vi "Launcher.vi"() -> ()   [LabVIEW 2023, in "Test Caller Actor.lvlib"]
uses:
  Test Caller Actor.lvlib
  Test Caller Actor/Test Caller Actor.lvclass
  Class Loader/Class Loader/Class Loader.lvclass
  Test Caller Actor/Test Caller Actor.lvclass/Test Caller Actor.ctl
  <vilib>/ActorFramework/Message Enqueuer/Message Enqueuer.lvclass/Message Enqueuer.ctl
  Test Caller Actor/Write Class Loader Enqueuer.vi
  <vilib>/ActorFramework/Message Enqueuer/Enqueue.vi
  <vilib>/ActorFramework/Stop Msg/Stop Msg.lvclass
  <vilib>/Utility/LVClass/Get LV Class Name.vi
  <resource>/AFDebug/Generate Trace for Message.vi
  <vilib>/ActorFramework/Message Priority Queue/Priority Enqueue.vi
  <vilib>/ActorFramework/Actor/Actor.lvclass
  C:/Program Files/National Instruments/LabVIEW 2023/vi.lib/LS Instruments AG/Async Methods Actor/Async Methods Actor/Async Methods Actor/Async Methods Actor.lvclass
  C:/Program Files/National Instruments/LabVIEW 2023/vi.lib/ActorFramework/Actor/Actor.lvclass
  C:/Projects/Shared Libraries/Class Loader/Class Loader/Class Loader/Class Loader.lvclass
  C:/Projects/Shared Libraries/Class Loader/Test Caller Actor/Test Caller Actor/Test Caller Actor.lvclass
  C:/Projects/Shared Libraries/Class Loader/Class Loader/Class Loader Interfaces/Class Loader Interfaces/Class Loader Interfaces.lvclass
panel:
  in  "Test Actor Number":i32=2
  in  "Stop Class Loader":bool
  out "error out":errorcluster
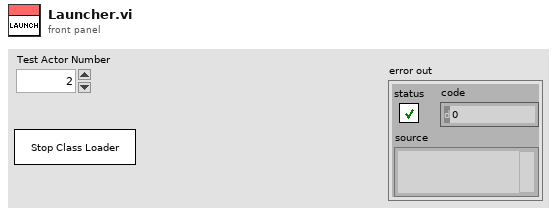
[diagram p1: front panel]
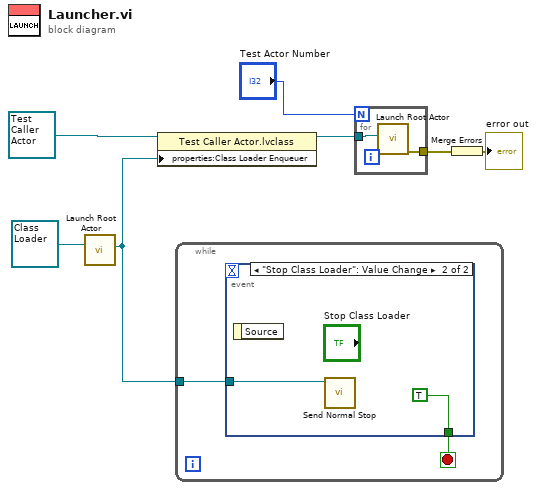
[diagram p0: block diagram]
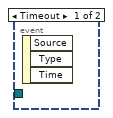
[diagram p2: hidden frame]
diagram:
  n1 = call <vilib>:"Launch Root Actor.vi"("Actor"=refnum<class "Class Loader.lvclass"> refnum ("Class Loader.lvlib:Class Loader.lvclass")) -> ("Actor's Enqueuer"=w2:refnum<class "Message Enqueuer.lvclass">)  [unwired: 9 in, 1 out]
  n2 = property class="Test Caller Actor.lvclass"(reference=refnum<class "Test Caller Actor.lvclass"> refnum ("Test Caller Actor.lvlib:Test Caller Actor.lvclass"), "properties:Class Loader Enqueuer"=w2) -> (reference out=w3:refnum<class "Test Caller Actor.lvclass">)  [unwired: 1 in, 1 out]
  n3 = while {
    tunnel: w2 -> [w9]
    stop <- w8 stop-if-true
    n4 = event shown="[1] \"Stop Class Loader\": Value Change" {
      selector: _ -> [_ _]
      dyn-events: _ -> [_ _]
      timeout: _ -> [_ _]
      tunnel: w9 -> [_ w11]
      tunnel: [_ TRUE] -> w8
      event Timeout {
        n5 = event-data() -> ()  [unwired: 1 in, 3 out]
      }
      event "Stop Class Loader": Value Change {
        n6 = event-data() -> ()  [unwired: 1 in, 1 out]
        n7 = call <vilib>:"Send Normal Stop.vi"("Message Enqueuer"=w11) -> ()  [unwired: 10 in, 1 out]
      }
    }
  }
  n8 = for {
    N: "Test Actor Number" -> [_]
    tunnel: [w13] -> w7
    tunnel: w3 -> [w12]
    n9 = call <vilib>:"Launch Root Actor.vi"("Actor"=w12) -> ("error out"=w13:errorcluster)  [unwired: 9 in, 1 out]
  }
  n10 = Merge Errors(w7) -> (→"error out":errorcluster)
